vi "mobileyelanepaser.vi"(11 "laneupdate":bool) -> (3 "update":bool)   [LabVIEW 2012]
uses:
  G_LCM.vi
  G_SEN.vi
panel:
  out "r":dbl
  in  "shift_c":dbl=-0.1
  in  "bias_b":dbl=0.005
  out "count":i32
  out "a":dbl
  out "b":dbl
  out "cl":dbl
  out "cr":dbl
  out "confidance_L":u8
  out "confidance_R":u8
  in  "bias_c":dbl=0.8
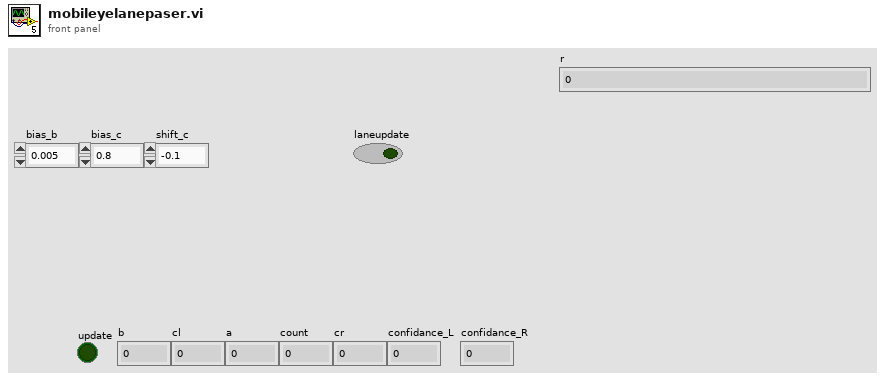
[diagram p1: front panel]
types:
  T1 = cluster{"hash":i64, "sys time":i64, "mobileye":u8[]}
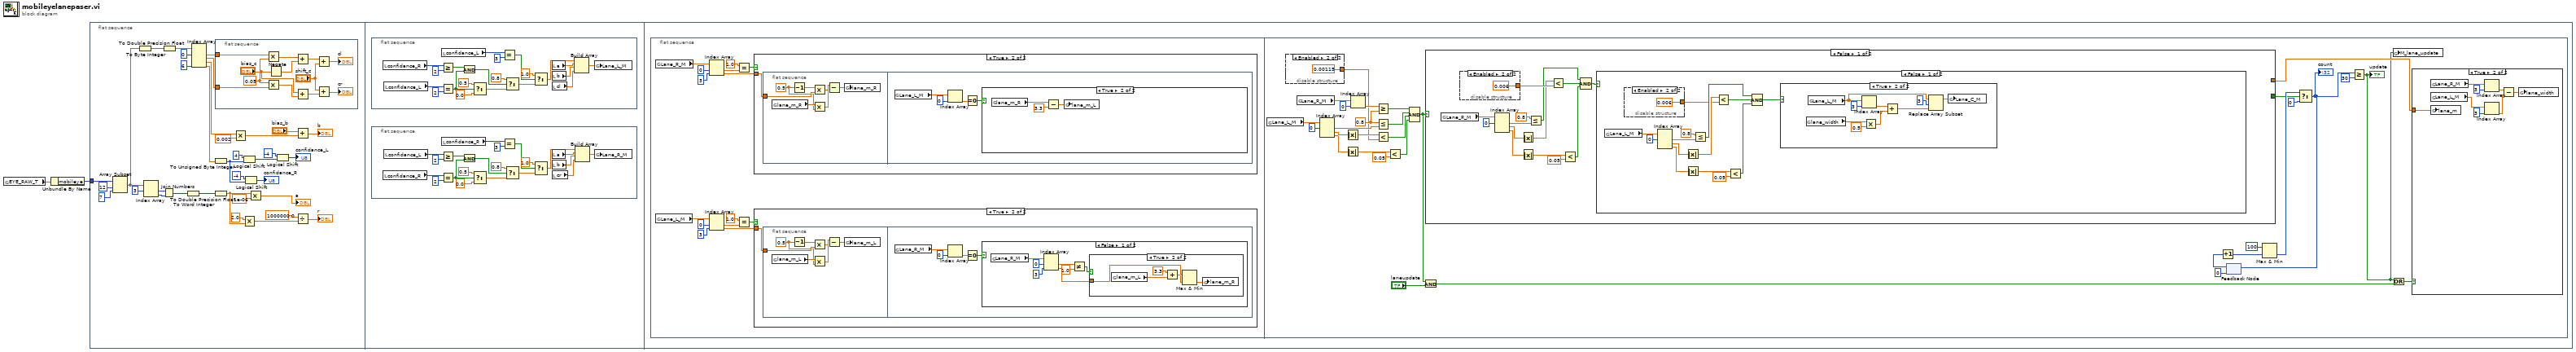
[diagram p0: block diagram]
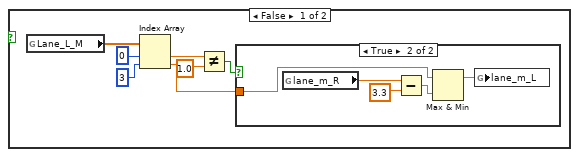
[diagram p3: hidden frame]
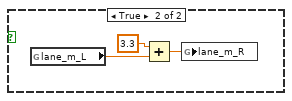
[diagram p7: hidden frame]
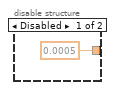
[diagram p8: hidden frame]
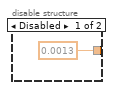
[diagram p10: hidden frame]
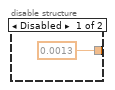
[diagram p11: hidden frame]
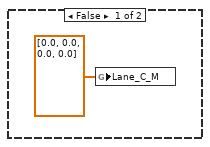
[diagram p12: hidden frame]
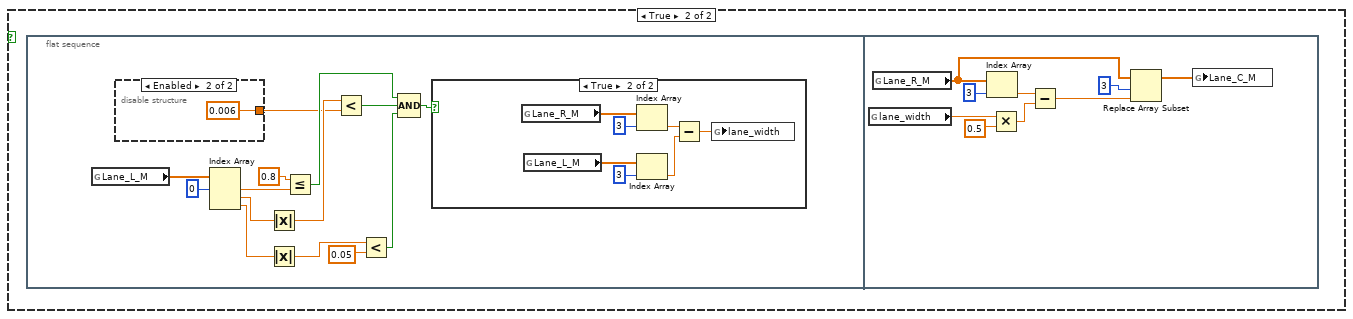
[diagram p13: hidden frame]
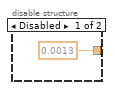
[diagram p14: hidden frame]
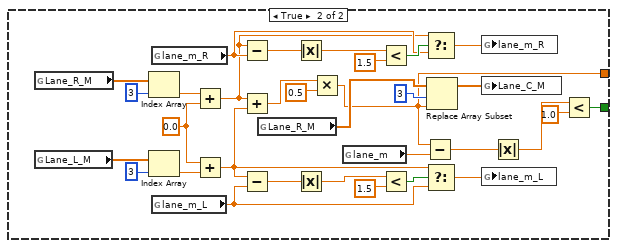
[diagram p16: hidden frame]
diagram:
  n1 = global read "G_LCM.vi" "EYE_RAW_T"() -> (w2:T1)
  n2 = Unbundle By Name(w2) -> ("mobileye"=w1:u8[])
  n3 = flat-sequence {
    tunnel: w1 -> [w15]
    frame #0 {
      n4 = Array Subset(array=w15, index=12, length=7) -> (w14:u8[])
      n5 = To Byte Integer(number=w14) -> (8bit integer=w34:i8[])
      n6 = Index Array(array=w14, index #1=3 ("index")) -> (element #1=w28:u8, element #2=w27:u8)  [unwired: 1 in]
      n7 = Join Numbers(hi=w28, lo=w27) -> ((hi.lo)=w26:u16)
      n8 = To Double Precision Float(number=w34) -> (double precision float=w33:dbl[])
      n9 = To Word Integer(number=w26) -> (16bit integer=w25:i16)
      n10 = Index Array(array=w33, index #1=0 ("index"), index #4=6 ("index")) -> (element #1=w32:dbl, element #2=w31:dbl, element #3=w30:dbl, element #4=w21:dbl)  [unwired: 2 in]
      n11 = To Unsigned Byte Integer(number=w21) -> (unsigned 8bit integer=w19:u8)
      n12 = To Double Precision Float(number=w25) -> (double precision float=w3:dbl)
      n13 = flat-sequence {
        tunnel: w32 -> [w49]
        tunnel: w31 -> [w48]
        frame #0 {
          w47 = 0.05 ("y")
          n14 = Multiply(x=w49, y=w47) -> (x*y=w45:dbl)
          n15 = Multiply(x=w47, y=w48) -> (x*y=w46:dbl)
          n16 = Negate(x="bias_c") -> (-x=w43:dbl)
          n17 = Add(x=w45, y=w43) -> (x+y=w42:dbl)
          n18 = Add(x="bias_c", y=w46) -> (x+y=w40:dbl)
          n19 = Add(x=w42, y="shift_c") -> (x+y=→"cl":dbl)
          n20 = Add(x="shift_c", y=w40) -> (x+y=→"cr":dbl)
        }
      }
      n21 = Multiply(x=w30, y=0.002) -> (x*y=w11:dbl)
      n22 = Logical Shift(y=i16 4, x=w19) -> (x << y=w17:u8)
      n23 = Multiply(x=2.0, y=w3) -> (x*y=w6:dbl)
      n24 = Logical Shift(y=i16 -4, x=w19) -> (x << y=→"confidance_R":u8)
      n25 = Multiply(x=w3, y=1e-06) -> (x*y=→"a":dbl)
      n26 = Logical Shift(y=i16 -4, x=w17) -> (x << y=→"confidance_L":u8)
      n27 = Add(x="bias_b", y=w11) -> (x+y=→"b":dbl)
      n28 = Divide(x=1000000.0 ("y"), y=w6) -> (x/y=→"r":dbl)
    }
    frame #1 {
      n29 = flat-sequence {
        frame #0 {
          n30 = local read "confidance_R"() -> (w90:u8)
          n31 = local read "confidance_L"() -> (w77:u8)
          n32 = Greater Or Equal?(x=w90, y=u8 2) -> (x >= y?=w72:bool)
          n33 = Equal?(x=w77, y=u8 2) -> (x = y?=w71:bool)
          n34 = local read "confidance_L"() -> (w88:u8)
          n35 = And(x=w72, y=w71) -> (x .and. y?=w80:bool)
          n36 = Select(t=0.5, s=w71, f=0.0) -> (s? t:f=w74:dbl)
          n37 = Equal?(x=w88, y=u8 3) -> (x = y?=w81:bool)
          n38 = Select(t=0.8, s=w80, f=w74) -> (s? t:f=w78:dbl)
          n39 = Select(t=1.0, s=w81, f=w78) -> (s? t:f=w83:dbl)
          n40 = local read "a"() -> (w85:dbl)
          n41 = local read "b"() -> (w86:dbl)
          n42 = local read "cl"() -> (w87:dbl)
          n43 = Build Array(w83, w85, w86, w87) -> (w84:dbl[])
          n44 = global write "G_SEN.vi" "Lane_L_M"(w84) -> ()
        }
      }
      n45 = flat-sequence {
        frame #0 {
          n46 = local read "confidance_R"() -> (w56:u8)
          n47 = local read "confidance_L"() -> (w69:u8)
          n48 = Greater Or Equal?(x=w69, y=u8 2) -> (x >= y?=w51:bool)
          n49 = Equal?(x=w56, y=u8 2) -> (x = y?=w50:bool)
          n50 = local read "confidance_R"() -> (w67:u8)
          n51 = And(x=w51, y=w50) -> (x .and. y?=w59:bool)
          n52 = Select(t=0.5, s=w50, f=0.0) -> (s? t:f=w53:dbl)
          n53 = Equal?(x=w67, y=u8 3) -> (x = y?=w61:bool)
          n54 = Select(t=0.8, s=w59, f=w53) -> (s? t:f=w57:dbl)
          n55 = Select(t=1.0, s=w61, f=w57) -> (s? t:f=w62:dbl)
          n56 = local read "a"() -> (w64:dbl)
          n57 = local read "b"() -> (w65:dbl)
          n58 = local read "cr"() -> (w66:dbl)
          n59 = Build Array(w62, w64, w65, w66) -> (w63:dbl[])
          n60 = global write "G_SEN.vi" "Lane_R_M"(w63) -> ()
        }
      }
    }
    frame #2 {
      n61 = flat-sequence {
        frame #0 {
          n62 = global read "G_SEN.vi" "Lane_R_M"() -> (w98:dbl[])
          n63 = global read "G_SEN.vi" "Lane_L_M"() -> (w105:dbl[])
          n64 = Index Array(array=w98, index #1=0 ("index"), index #2=3 ("index")) -> (element #1=w97:dbl, element #2=w101:dbl)
          n65 = Index Array(array=w105, index #1=0 ("index"), index #2=3 ("index")) -> (element #1=w93:dbl, element #2=w102:dbl)
          n66 = Equal?(x=1.0, y=w97) -> (x = y?=w95:bool)
          n67 = Equal?(x=1.0, y=w93) -> (x = y?=w92:bool)
          n68 = case shown="True" w95 {
            tunnel: w101 -> [_ w106]
            frame False {
            }
            frame True {
              n69 = flat-sequence {
                tunnel: w106 -> [w112]
                frame #0 {
                  w108 = 0.5 ("y")
                  n70 = global read "G_SEN.vi" "lane_m_R"() -> (w113:dbl)
                  n71 = Decrement(x=w108) -> (x-1=w107:dbl)
                  n72 = Multiply(x=w107, y=w112) -> (x*y=w110:dbl)
                  n73 = Multiply(x=w113, y=w108) -> (x*y=w111:dbl)
                  n74 = Subtract(x=w111, y=w110) -> (x-y=w109:dbl)
                  n75 = global write "G_SEN.vi" "lane_m_R"(w109) -> ()
                }
                frame #1 {
                  n76 = global read "G_SEN.vi" "Lane_L_M"() -> (w116:dbl[])
                  n77 = Index Array(array=w116, index=0) -> (element=w115:dbl)
                  n78 = Equal To 0?(x=w115) -> (x = 0?=w114:bool)
                  n79 = case shown="True" w114 {
                    frame False {
                      n80 = global read "G_SEN.vi" "Lane_L_M"() -> (w119:dbl[])
                      n81 = Index Array(array=w119, index #1=0 ("index"), index #2=3 ("index")) -> (element #1=w120:dbl, element #2=w124:dbl)
                      n82 = Not Equal?(x=w120, y=1.0) -> (x != y?=w122:bool)
                      n83 = case shown="True" w122 {
                        tunnel: w124 -> [_ w129]
                        frame False {
                        }
                        frame True {
                          n84 = global read "G_SEN.vi" "lane_m_R"() -> (w127:dbl)
                          n85 = Subtract(x=w127, y=3.3) -> (x-y=w128:dbl)
                          n86 = Max & Min(x=w129, y=w128) -> (max(x,y)=w125:dbl)  [unwired: 1 out]
                          n87 = global write "G_SEN.vi" "lane_m_L"(w125) -> ()
                        }
                      }
                    }
                    frame True {
                      n88 = global read "G_SEN.vi" "lane_m_R"() -> (w132:dbl)
                      n89 = Subtract(x=w132, y=3.3) -> (x-y=w130:dbl)
                      n90 = global write "G_SEN.vi" "lane_m_L"(w130) -> ()
                    }
                  }
                }
              }
            }
          }
          n91 = case shown="True" w92 {
            tunnel: w102 -> [_ w133]
            frame False {
            }
            frame True {
              n92 = flat-sequence {
                tunnel: w133 -> [w139]
                frame #0 {
                  w135 = 0.5 ("y")
                  n93 = global read "G_SEN.vi" "lane_m_L"() -> (w140:dbl)
                  n94 = Decrement(x=w135) -> (x-1=w134:dbl)
                  n95 = Multiply(x=w134, y=w139) -> (x*y=w137:dbl)
                  n96 = Multiply(x=w140, y=w135) -> (x*y=w138:dbl)
                  n97 = Subtract(x=w138, y=w137) -> (x-y=w136:dbl)
                  n98 = global write "G_SEN.vi" "lane_m_L"(w136) -> ()
                }
                frame #1 {
                  n99 = global read "G_SEN.vi" "Lane_R_M"() -> (w144:dbl[])
                  n100 = Index Array(array=w144, index=0) -> (element=w142:dbl)
                  n101 = Equal To 0?(x=w142) -> (x = 0?=w141:bool)
                  n102 = case shown="False" w141 {
                    frame False {
                      n103 = global read "G_SEN.vi" "Lane_R_M"() -> (w150:dbl[])
                      n104 = Index Array(array=w150, index #1=0 ("index"), index #2=3 ("index")) -> (element #1=w149:dbl, element #2=w145:dbl)
                      n105 = Not Equal?(x=w149, y=1.0) -> (x != y?=w147:bool)
                      n106 = case shown="True" w147 {
                        tunnel: w145 -> [_ w154]
                        frame False {
                        }
                        frame True {
                          n107 = global read "G_SEN.vi" "lane_m_L"() -> (w155:dbl)
                          n108 = Add(x=3.3 ("y"), y=w155) -> (x+y=w153:dbl)
                          n109 = Max & Min(x=w154, y=w153) -> (min(x,y)=w152:dbl)  [unwired: 1 out]
                          n110 = global write "G_SEN.vi" "lane_m_R"(w152) -> ()
                        }
                      }
                    }
                    frame True {
                      n111 = global read "G_SEN.vi" "lane_m_L"() -> (w157:dbl)
                      n112 = Add(x=3.3 ("y"), y=w157) -> (x+y=w159:dbl)
                      n113 = global write "G_SEN.vi" "lane_m_R"(w159) -> ()
                    }
                  }
                }
              }
            }
          }
        }
        frame #1 {
          w188 = 0.8 ("y")
          n114 = global read "G_SEN.vi" "Lane_L_M"() -> (w186:dbl[])
          n115 = disable-structure shown="Enabled" {
            disable-tunnel: [0.0005 0.00115] -> w168
            frame Disabled {
            }
            frame Enabled {
            }
          }
          n116 = global read "G_SEN.vi" "Lane_R_M"() -> (w183:dbl[])
          n117 = Index Array(array=w186, index #1=0 ("index")) -> (element #1=w189:dbl, element #2=w182:dbl, element #3=w165:dbl)  [unwired: 2 in]
          n118 = Absolute Value(x=w182) -> (abs(x)=w181:dbl)
          n119 = Absolute Value(x=w165) -> (abs(x)=w164:dbl)
          n120 = Index Array(array=w183, index=0) -> (element=w187:dbl)
          n121 = Greater Or Equal?(x=w187, y=w188) -> (x >= y?=w190:bool)
          n122 = Less Or Equal?(x=w188, y=w189) -> (x <= y?=w191:bool)
          n123 = Less?(x=w181, y=w168) -> (x < y?=w180:bool)
          n124 = Less?(x=w164, y=0.05) -> (x < y?=w162:bool)
          n125 = Compound Arithmetic op=AND(w190, w191, w180, w162) -> (w160:bool)
          n126 = And(x=w160, y="laneupdate") -> (x .and. y?=w166:bool)
          n127 = case shown="False" w160 {
            tunnel: [_ w285] -> w170
            tunnel: [_ w276] -> w171
            frame False {
              n128 = global read "G_SEN.vi" "Lane_R_M"() -> (w215:dbl[])
              n129 = disable-structure shown="Enabled" {
                disable-tunnel: [0.0013 0.006] -> w213
                frame Disabled {
                }
                frame Enabled {
                }
              }
              n130 = Index Array(array=w215, index #1=0 ("index")) -> (element #1=w212:dbl, element #2=w208:dbl, element #3=w203:dbl)  [unwired: 2 in]
              n131 = Absolute Value(x=w208) -> (abs(x)=w207:dbl)
              n132 = Absolute Value(x=w203) -> (abs(x)=w205:dbl)
              n133 = Less Or Equal?(x=0.8 ("y"), y=w212) -> (x <= y?=w211:bool)
              n134 = Less?(x=w207, y=w213) -> (x < y?=w210:bool)
              n135 = Less?(x=w205, y=0.05) -> (x < y?=w202:bool)
              n136 = Compound Arithmetic op=AND(w211, w210, w202) -> (w209:bool)
              n137 = case shown="False" w209 {
                frame False {
                  n138 = global read "G_SEN.vi" "Lane_L_M"() -> (w226:dbl[])
                  n139 = disable-structure shown="Enabled" {
                    disable-tunnel: [0.0013 0.006] -> w222
                    frame Disabled {
                    }
                    frame Enabled {
                    }
                  }
                  n140 = Index Array(array=w226, index #1=0 ("index")) -> (element #1=w229:dbl, element #2=w224:dbl, element #3=w219:dbl)  [unwired: 2 in]
                  n141 = Absolute Value(x=w224) -> (abs(x)=w223:dbl)
                  n142 = Absolute Value(x=w219) -> (abs(x)=w221:dbl)
                  n143 = Less Or Equal?(x=0.8 ("y"), y=w229) -> (x <= y?=w230:bool)
                  n144 = Less?(x=w223, y=w222) -> (x < y?=w231:bool)
                  n145 = Less?(x=w221, y=0.05) -> (x < y?=w218:bool)
                  n146 = Compound Arithmetic op=AND(w230, w231, w218) -> (w225:bool)
                  n147 = case shown="True" w225 {
                    frame False {
                      n148 = global write "G_SEN.vi" "Lane_C_M"(dbl[] [0.0, 0.0, 0.0, 0.0] ("Lane_C_M")) -> ()
                    }
                    frame True {
                      n149 = global read "G_SEN.vi" "lane_width"() -> (w240:dbl)
                      n150 = global read "G_SEN.vi" "Lane_L_M"() -> (w236:dbl[])
                      n151 = Index Array(array=w236, index=3) -> (element=w241:dbl)
                      n152 = Multiply(x=w240, y=0.5) -> (x*y=w238:dbl)
                      n153 = Add(x=w241, y=w238) -> (x+y=w237:dbl)
                      n154 = Replace Array Subset(array=w236, new element=w237, index=3) -> (w235:dbl[])
                      n155 = global write "G_SEN.vi" "Lane_C_M"(w235) -> ()
                    }
                  }
                }
                frame True {
                  n156 = flat-sequence {
                    frame #0 {
                      n157 = global read "G_SEN.vi" "Lane_L_M"() -> (w252:dbl[])
                      n158 = disable-structure shown="Enabled" {
                        disable-tunnel: [0.0013 0.006] -> w248
                        frame Disabled {
                        }
                        frame Enabled {
                        }
                      }
                      n159 = Index Array(array=w252, index #1=0 ("index")) -> (element #1=w255:dbl, element #2=w251:dbl, element #3=w245:dbl)  [unwired: 2 in]
                      n160 = Absolute Value(x=w251) -> (abs(x)=w250:dbl)
                      n161 = Absolute Value(x=w245) -> (abs(x)=w247:dbl)
                      n162 = Less Or Equal?(x=0.8 ("y"), y=w255) -> (x <= y?=w256:bool)
                      n163 = Less?(x=w250, y=w248) -> (x < y?=w257:bool)
                      n164 = Less?(x=w247, y=0.05) -> (x < y?=w244:bool)
                      n165 = Compound Arithmetic op=AND(w256, w257, w244) -> (w249:bool)
                      n166 = case shown="True" w249 {
                        frame False {
                        }
                        frame True {
                          n167 = global read "G_SEN.vi" "Lane_R_M"() -> (w261:dbl[])
                          n168 = global read "G_SEN.vi" "Lane_L_M"() -> (w263:dbl[])
                          n169 = Index Array(array=w261, index=3) -> (element=w264:dbl)
                          n170 = Index Array(array=w263, index=3) -> (element=w265:dbl)
                          n171 = Subtract(x=w264, y=w265) -> (x-y=w266:dbl)
                          n172 = global write "G_SEN.vi" "lane_width"(w266) -> ()
                        }
                      }
                    }
                    frame #1 {
                      n173 = global read "G_SEN.vi" "lane_width"() -> (w270:dbl)
                      n174 = global read "G_SEN.vi" "Lane_R_M"() -> (w274:dbl[])
                      n175 = Index Array(array=w274, index=3) -> (element=w269:dbl)
                      n176 = Multiply(x=w270, y=0.5) -> (x*y=w272:dbl)
                      n177 = Subtract(x=w269, y=w272) -> (x-y=w273:dbl)
                      n178 = Replace Array Subset(array=w274, new element=w273, index=3) -> (w275:dbl[])
                      n179 = global write "G_SEN.vi" "Lane_C_M"(w275) -> ()
                    }
                  }
                }
              }
            }
            frame True {
              w280 = 0.0 ("y")
              n180 = global read "G_SEN.vi" "Lane_R_M"() -> (w306:dbl[])
              n181 = global read "G_SEN.vi" "Lane_L_M"() -> (w295:dbl[])
              n182 = Index Array(array=w306, index=3) -> (element=w284:dbl)
              n183 = Index Array(array=w295, index=3) -> (element=w282:dbl)
              n184 = global read "G_SEN.vi" "lane_m_R"() -> (w301:dbl)
              n185 = global read "G_SEN.vi" "lane_m_L"() -> (w300:dbl)
              n186 = Add(x=w284, y=w280) -> (x+y=w283:dbl)
              n187 = Add(x=w280, y=w282) -> (x+y=w281:dbl)
              n188 = Subtract(x=w283, y=w301) -> (x-y=w305:dbl)
              n189 = Add(x=w283, y=w281) -> (x+y=w292:dbl)
              n190 = Subtract(x=w281, y=w300) -> (x-y=w296:dbl)
              n191 = global read "G_SEN.vi" "Lane_R_M"() -> (w277:dbl[])
              n192 = Absolute Value(x=w305) -> (abs(x)=w304:dbl)
              n193 = Absolute Value(x=w296) -> (abs(x)=w297:dbl)
              n194 = Multiply(x=w292, y=0.5) -> (x*y=w276:dbl)
              n195 = global read "G_SEN.vi" "lane_m"() -> (w289:dbl)
              n196 = Less?(x=w304, y=1.5) -> (x < y?=w302:bool)
              n197 = Less?(x=w297, y=1.5) -> (x < y?=w299:bool)
              n198 = Subtract(x=w276, y=w289) -> (x-y=w286:dbl)
              n199 = Select(t=w283, s=w302, f=w301) -> (s? t:f=w291:dbl)
              n200 = Select(t=w281, s=w299, f=w300) -> (s? t:f=w290:dbl)
              n201 = Replace Array Subset(array=w277, new element=w276, index=3) -> (w279:dbl[])
              n202 = global write "G_SEN.vi" "lane_m_R"(w291) -> ()
              n203 = global write "G_SEN.vi" "Lane_C_M"(w279) -> ()
              n204 = global write "G_SEN.vi" "lane_m_L"(w290) -> ()
              n205 = Absolute Value(x=w286) -> (abs(x)=w287:dbl)
              n206 = Less?(x=w287, y=1.0) -> (x < y?=w285:bool)
            }
          }
          n207 = feedback #1(0) -> (w178:i32)
          n208 = Increment(x=w178) -> (x+1=w174:i32)
          n209 = Max & Min(x=100, y=w174) -> (min(x,y)=w173:i32)  [unwired: 1 out]
          n210 = Select(t=w173, s=w170, f=0) -> (s? t:f=w176:i32)
          "count" <- w176
          n211 = feedback-in #1(w176) -> ()
          n212 = Greater Or Equal?(x=w176, y=30) -> (x >= y?=w167:bool)
          "update" <- w167
          n213 = Or(x=w167, y=w166) -> (x .or. y?=w169:bool)
          n214 = global write "G_SEN.vi" "M_lane_update"(w167) -> ()
          n215 = case shown="True" w169 {
            tunnel: w171 -> [_ w194]
            frame False {
            }
            frame True {
              n216 = global read "G_SEN.vi" "Lane_R_M"() -> (w201:dbl[])
              n217 = global read "G_SEN.vi" "Lane_L_M"() -> (w198:dbl[])
              n218 = global write "G_SEN.vi" "lane_m"(w194) -> ()
              n219 = Index Array(array=w201, index=3) -> (element=w197:dbl)
              n220 = Index Array(array=w198, index=3) -> (element=w196:dbl)
              n221 = Subtract(x=w197, y=w196) -> (x-y=w195:dbl)
              n222 = global write "G_SEN.vi" "lane_width"(w195) -> ()
            }
          }
        }
      }
    }
  }
